vi "Autoshift and Fall preventor Test.vi"() -> ()   [LabVIEW 2018]
uses:
  <vilib>/Rock Robotics/WPI/ThirdParty/Phoenix-LabVIEW/Pigeon IMU/CTRE_PigeonIMU_GetYPR.vi
  <vilib>/addons/control/pid/NI_PID_pid.lvlib
  <vilib>/addons/control/pid/pid.llb/PID (DBL).vi
panel:
  out "Power":dbl
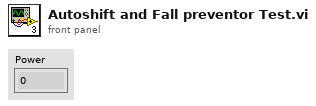
[diagram p1: front panel]
types:
  T1 = cluster{"proportional gain (Kc)":dbl, "integral time (Ti, min)":dbl, "derivative time (Td, min)":dbl}
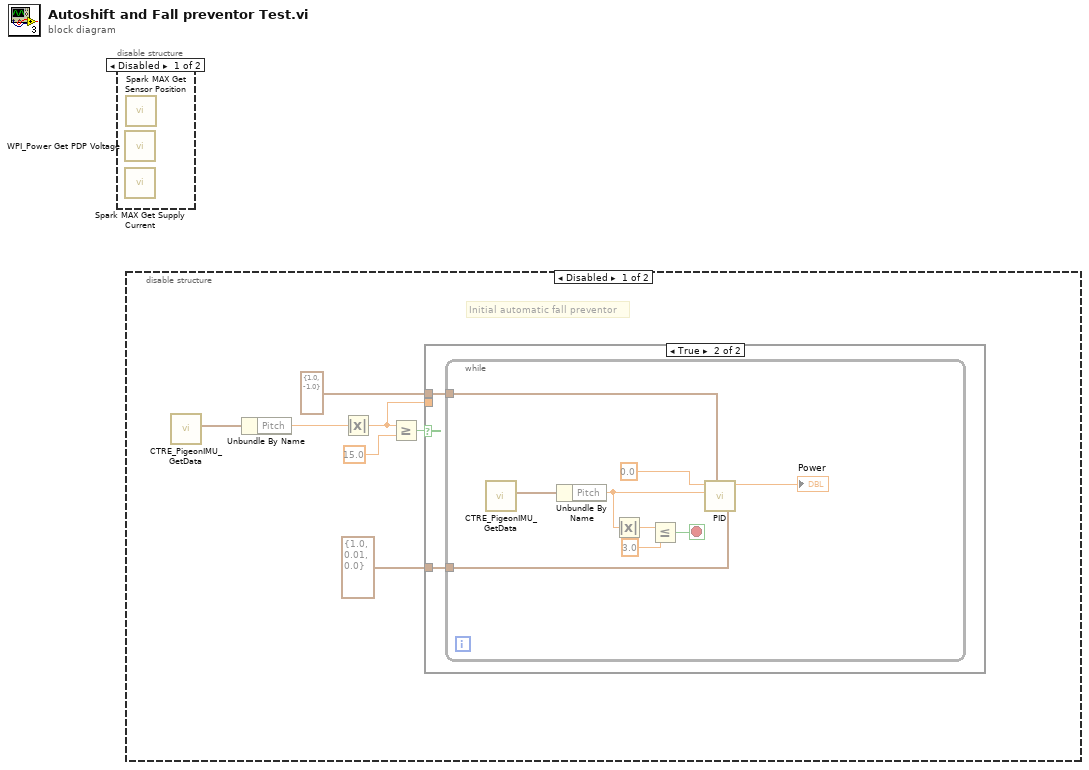
[diagram p0: block diagram]
diagram:
  n1 = disable-structure shown="Disabled" {
    frame Disabled {
      n2 = call <vilib>:"WPI_Power Get PDP Voltage.vi"() -> ()  [unwired: 14 in, 2 out]
      n3 = call <vilib>:"Spark MAX Get Supply Current.vi"() -> ()  [unwired: 8 in, 4 out]
      n4 = call <vilib>:"Spark MAX Get Sensor Position.vi"() -> ()  [unwired: 8 in, 4 out]
    }
    frame Enabled {
    }
  }
  n5 = disable-structure shown="Disabled" {
    frame Disabled {
      # "Initial automatic fall preventor"
      n6 = call-poly <vilib>:"CTRE_PigeonIMU_GetData.vi"() -> ("Yaw Pitch Roll"=w7:cluster{"Yaw":dbl, "Pitch":dbl, "Roll":dbl})  [unwired: 9 in, 2 out]
      n7 = Unbundle By Name(w7) -> ("Pitch"=w6:dbl)
      n8 = Absolute Value(x=w6) -> (abs(x)=w3:dbl)
      n9 = Greater Or Equal?(x=w3, y=15.0) -> (x >= y?=w4:bool)
      n10 = case shown="True" w4 {
        tunnel: w3 -> [_ _]
        tunnel: T1 {"proportional gain (Kc)"=1.0, "integral time (Ti, min)"=0.01, "derivative time (Td, min)"=0.0} ("PID gains") -> [_ w9]
        tunnel: cluster{"output high":dbl, "output low":dbl} {"output high"=1.0, "output low"=-1.0} ("output range") -> [_ w8]
        frame False {
        }
        frame True {
          n11 = while {
            tunnel: w9 -> [w16]
            tunnel: w8 -> [w15]
            stop <- w13 stop-if-true
            n12 = call-poly <vilib>:"CTRE_PigeonIMU_GetData.vi"() -> ("Yaw Pitch Roll"=w17:cluster{"Yaw":dbl, "Pitch":dbl, "Roll":dbl})  [unwired: 9 in, 2 out]
            n13 = Unbundle By Name(w17) -> ("Pitch"=w14:dbl)
            n14 = Absolute Value(x=w14) -> (abs(x)=w12:dbl)
            n15 = Less Or Equal?(x=w12, y=3.0) -> (x <= y?=w13:bool)
            n16 = call-poly <vilib>:"PID.vi"("output range"=w15, "PID gains"=w16, "process variable"=w14, "setpoint"=0.0) -> ("output"=→"Power":dbl)  [unwired: 6 in, 1 out]
          }
        }
      }
    }
    frame Enabled {
    }
  }
